vi "ReferencedVariables_ReadWriteReferencedVariable_6x8x6.vi"(0 "reference in":refnum<class>, 2 "ReplaceWithtypeDef":dbl, 5 "error in (no error)":errorcluster) -> (14 "reference out":refnum<class>, 19 "error out":errorcluster)   [LabVIEW 2014]
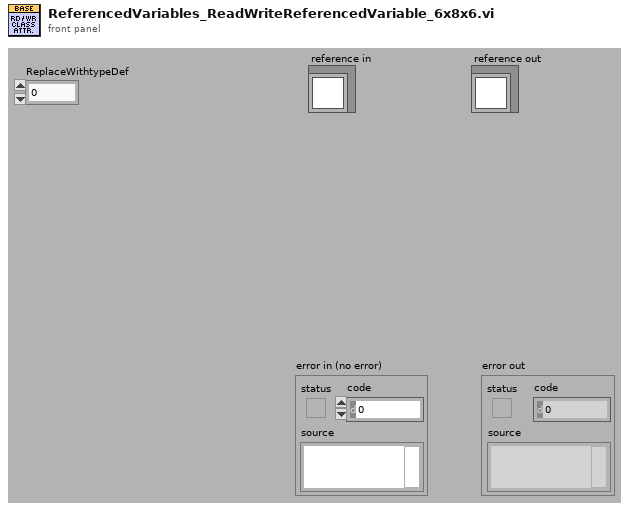
[diagram p1: front panel]
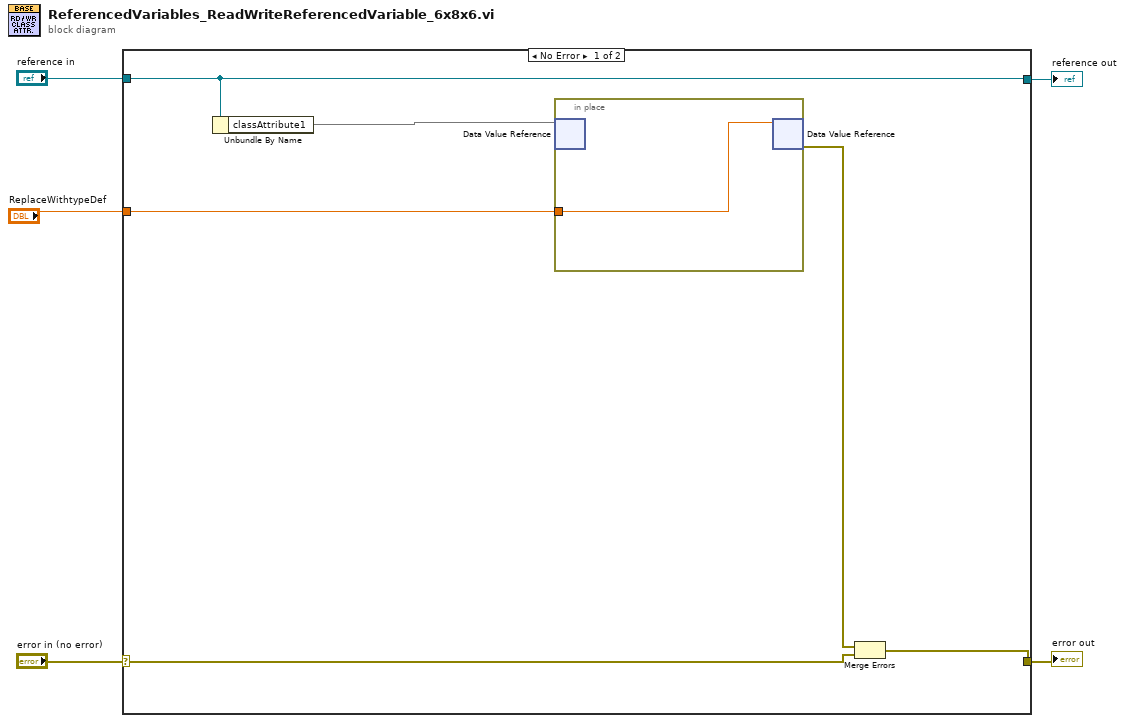
[diagram p0: block diagram]
diagram:
  n1 = case shown="No Error" "error in (no error)" {
    selector: "error in (no error)" -> [w7 w14]
    tunnel: [w10 w14] -> w4
    tunnel: [w9 w13] -> w2
    tunnel: "reference in" -> [w9 w13]
    tunnel: "ReplaceWithtypeDef" -> [w8 _]
    frame No Error {
      n2 = Unbundle By Name(w9) -> ("classAttribute1"=w6)
      n3 = in-place {
        in-place-border: w8 -> [w12]
        n4 = in-place-dvr #1(w6) -> ()  [unwired: 2 out]
        n5 = in-place-dvr #1(w12) -> (w11:errorcluster)  [unwired: 1 out]
      }
      n6 = Merge Errors(w11, w7) -> (w10:errorcluster)
    }
    frame Error {
    }
  }
  "error out" <- w4
  "reference out" <- w2
